vi "SmartSEM Remote API FIB HV offset removal.vi"(9 "Max offset threshold (V)":sgl=100.0, 11 "Api":refnum<k7>(container)) -> (1 "FIB HV matched":bool, 3 "Max HV offset (V)":sgl)   [LabVIEW 2018]
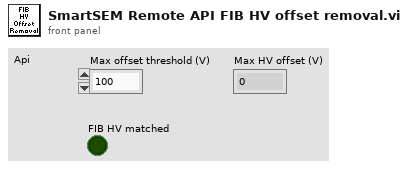
[diagram p1: front panel]
types:
  T1 = cluster{"Filament (A)":sgl, "Accelerator Target (V)":sgl, "Accelerator Actual (V)":sgl, "Extrator Target (V)":sgl, "Extrator Actual (V)":sgl, "Emission Target (uA)":sgl, "Emission Actual (uA)":sgl, "Suppressor (V)":sgl, "Faraday I (nA)":sgl, "Lens1 Target (V)":sgl, "Lens1 Actual (V)":sgl, "Lens2 Target (V)":sgl, "Lens2 Actual (V)":sgl, "Gun Vac (Torr)":sgl, "Column Vac (Torr)":sgl, "Tip Lifetime (uAhr)":sgl}
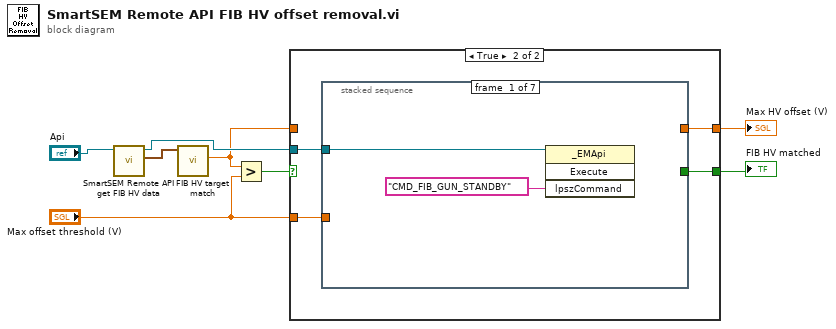
[diagram p0: block diagram]
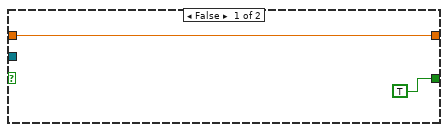
[diagram p2: hidden frame]
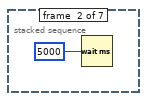
[diagram p3: hidden frame]
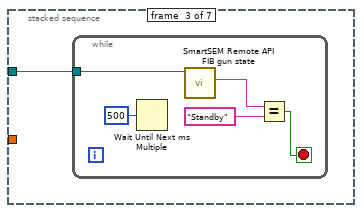
[diagram p4: hidden frame]
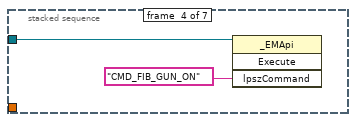
[diagram p5: hidden frame]
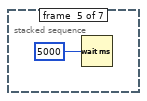
[diagram p6: hidden frame]
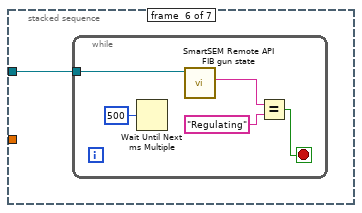
[diagram p7: hidden frame]
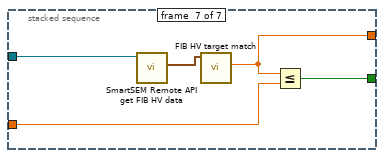
[diagram p8: hidden frame]
diagram:
  n1 = call "SmartSEM Remote API get FIB HV data.vi"("Api in"="Api") -> ("Capella HV Data Output"=w8:T1, "Api out"=w6:refnum<k7>)  [unwired: 7 in, 2 out]
  n2 = call "FIB HV target match.vi"("Capella HV Data Output"=w8) -> ("Max absolute error (V)"=w1:sgl)  [unwired: 5 in, 5 out]
  n3 = Greater?(x=w1, y="Max offset threshold (V)") -> (0:w4:bool)
  n4 = case shown="True" w4 {
    tunnel: w6 -> [_ w14]
    tunnel: "Max offset threshold (V)" -> [_ w13]
    tunnel: [TRUE w12] -> w3
    tunnel: [w9 w11] -> w2
    tunnel: w1 -> [w9 _]
    frame False {
    }
    frame True {
      n5 = stacked-sequence {
        tunnel: w14 -> [w15 _ w18 w24 _ w27 w37]
        tunnel: w13 -> [_ _ _ _ _ _ w36]
        tunnel: [_ _ _ _ _ _ w34] -> w12
        tunnel: [_ _ _ _ _ _ w33] -> w11
        frame #0 {
          n6 = invoke class="_EMApi" method="Execute"(reference=w15, "lpszCommand"="CMD_FIB_GUN_STANDBY") -> ()  [unwired: 2 in, 4 out]
        }
        frame #1 {
          n7 = Wait (ms)(milliseconds to wait=u32 5000) -> ()  [unwired: 1 out]
        }
        frame #2 {
          n8 = while {
            tunnel: w18 -> [w23]
            stop <- w20 stop-if-true
            n9 = Wait Until Next ms Multiple(millisecond multiple=u32 500) -> ()  [unwired: 1 out]
            n10 = call "SmartSEM Remote API FIB gun state.vi"("Api"=w23) -> ("FIB Gun State"=w22:string)  [unwired: 8 in, 2 out]
            n11 = Equal?(x=w22, y="Standby" ("FIB Gun State")) -> (x = y?=w20:bool)
          }
        }
        frame #3 {
          n12 = invoke class="_EMApi" method="Execute"(reference=w24, "lpszCommand"="CMD_FIB_GUN_ON") -> ()  [unwired: 2 in, 4 out]
        }
        frame #4 {
          n13 = Wait (ms)(milliseconds to wait=u32 5000) -> ()  [unwired: 1 out]
        }
        frame #5 {
          n14 = while {
            tunnel: w27 -> [w32]
            stop <- w29 stop-if-true
            n15 = Wait Until Next ms Multiple(millisecond multiple=u32 500) -> ()  [unwired: 1 out]
            n16 = call "SmartSEM Remote API FIB gun state.vi"("Api"=w32) -> ("FIB Gun State"=w31:string)  [unwired: 8 in, 2 out]
            n17 = Equal?(x=w31, y="Regulating" ("FIB Gun State")) -> (x = y?=w29:bool)
          }
        }
        frame #6 {
          n18 = call "SmartSEM Remote API get FIB HV data.vi"("Api in"=w37) -> ("Capella HV Data Output"=w35:T1)  [unwired: 7 in, 3 out]
          n19 = call "FIB HV target match.vi"("Capella HV Data Output"=w35) -> ("Max absolute error (V)"=w33:sgl)  [unwired: 5 in, 5 out]
          n20 = Less Or Equal?(x=w33, y=w36) -> (x <= y?=w34:bool)
        }
      }
    }
  }
  "FIB HV matched" <- w3
  "Max HV offset (V)" <- w2
